vi "Get Status.vi"(8 "error in (no error)":errorcluster, 11 "DPO4104 in":refnum<class "DPO4104.lvclass">) -> (0 "error out":errorcluster, 2 "Status Array":bool[](array[boolean]), 3 "DPO4104 out":refnum<class "DPO4104.lvclass">)   [LabVIEW 2018, in "DPO4104.lvlib" / "DPO4104.lvclass"]
doc: "This Override method is used to get the Oscope instrument status. The status data MUST be formatted into the 'Status Array' indicator as 1D array of boolean data ."
uses:
  DPO4104.lvclass
  PPLs/Oscilloscope/Parent/Oscilloscope.lvlibp/Oscilloscope.lvclass
  C:/Projects/LabVIEW/PPLs/Oscilloscope/Parent/Oscilloscope.lvlibp/Oscilloscope.lvclass
panel:
  # "OPC - Operation Complete"
  # "RQC - Request Control"
  # "QYE  - Query Error"
  # "DDE - DEvice Error"
  # "EXE - Execution Error"
  # "CME - Command Error"
  # "URQ - User  Request"
  # "PON - Power On"
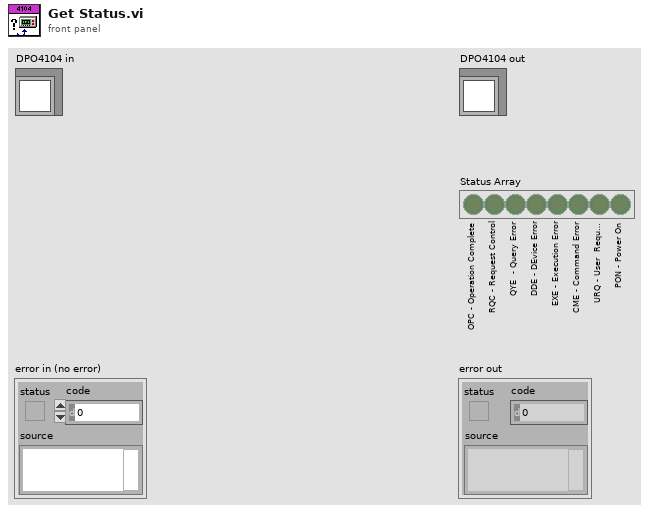
[diagram p1: front panel]
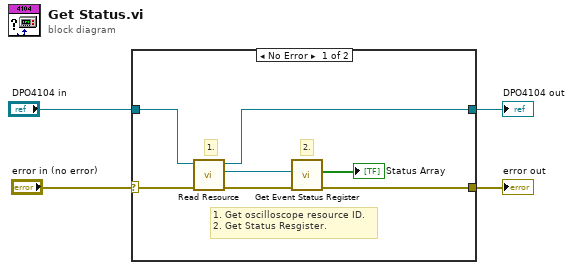
[diagram p0: block diagram]
diagram:
  n1 = case shown="No Error" "error in (no error)" {
    selector: "error in (no error)" -> [w5 w12]
    tunnel: [w6 w12] -> w3
    tunnel: [w10 w13] -> w1
    tunnel: "DPO4104 in" -> [w11 w13]
    frame No Error {
      # "2."
      # "1."
      # "1. Get oscilloscope resource ID.\n2. Get Status Resgister."
      n2 = call "Read Resource.vi"("error in (no error)"=w5, "Oscilloscope in"=w11) -> ("error out"=w8:errorcluster, "Resource"=w9:refnum<visa-resource-name>, "Oscilloscope out"=w10:refnum<class "DPO4104.lvclass">)  [unwired: 7 in]
      n3 = call "Get Event Status Register.vi"("error in (no error)"=w8, "VISA resource name"=w9) -> ("error out"=w6:errorcluster, "Event Status Register"=→"Status Array":bool[])  [unwired: 7 in, 1 out]
    }
    frame Error {
    }
  }
  "error out" <- w3
  "DPO4104 out" <- w1
